vi "test-trajectory-json.vi"(8 "error in (no error)":errorcluster) -> (0 "error out 2":errorcluster, 3 "ALL TESTS PASSED":bool)   [LabVIEW 2019]
uses:
  <vilib>/Rock Robotics/WPI/ThirdParty/JAS_Junk/TrajLib/POSE2D.ctl
  <vilib>/Rock Robotics/WPI/ThirdParty/JAS_Junk/TrajLib/TRANSLATION2D.ctl
  <vilib>/Rock Robotics/WPI/ThirdParty/JAS_Junk/TrajLib/ROTATION2D.ctl
  <vilib>/Rock Robotics/WPI/ThirdParty/JAS_Junk/TrajLib/TRAJECTORY.ctl
  <vilib>/Rock Robotics/WPI/ThirdParty/JAS_Junk/TrajLib/TRAJ_STATE.ctl
  <vilib>/Rock Robotics/SystemInterfaces/NetworkCommunication/NetComm_UsageReport_report.vi
  <vilib>/Rock Robotics/WPI/ThirdParty/JAS_Junk/TrajLib/DiffDriveKinematicsConstraint_New.vi
  TrajectoryState_AlmostEquals.vi
  <vilib>/Rock Robotics/WPI/ThirdParty/JAS_Junk/TrajLib/Util_ApproxEquals.vi
  Pose_AlmostEquals.vi
  Translation_AlmostEquals.vi
  Rotation_AlmostEquals.vi
  <vilib>/Rock Robotics/WPI/ThirdParty/JAS_Junk/TrajLib/Util_CalcDist.vi
  <vilib>/Rock Robotics/WPI/ThirdParty/JAS_Junk/TrajLib/Util_LibraryGlobals.vi
  <vilib>/Rock Robotics/WPI/ThirdParty/JAS_Junk/TrajLib/Trajectory_Library.lvlib
panel:
  out "Read Full \nFilename":string
  out "Write Full \nFilename":string
  in  "Tolerance":dbl=1e-06 format="%#_13g"
  out "outTRAJECTORY":T1 {"States"."POSE"."ROTATION"."SIN" format="%13.4f"; "States"."POSE"."ROTATION"."COS" format="%13.4f"; "States"."POSE"."ROTATION"."VALUE" format="%13.4f"; "States"."POSE"."TRANSLATION"."Y" format="%14.3f"; "States"."POSE"."TRANSLATION"."X" format="%14.3f"; "TotalTImeSecs" format="%20.3f"}
  out "TRAJECTORY":T1 {"States"."POSE"."ROTATION"."SIN" format="%13.4f"; "States"."POSE"."ROTATION"."COS" format="%13.4f"; "States"."POSE"."ROTATION"."VALUE" format="%13.4f"; "States"."POSE"."TRANSLATION"."Y" format="%14.3f"; "States"."POSE"."TRANSLATION"."X" format="%14.3f"; "TotalTImeSecs" format="%20.3f"}
  out "Equals":bool
  out "Read JSON":errorcluster
  out "Create JSON":errorcluster
  out "Waypoints":T3[](array[typedef]) {"ROTATION"."SIN" format="%13.4f"; "ROTATION"."COS" format="%13.4f"; "ROTATION"."VALUE" format="%13.4f"; "TRANSLATION"."Y" format="%14.3f"; "TRANSLATION"."X" format="%14.3f"}
  out "error out":errorcluster
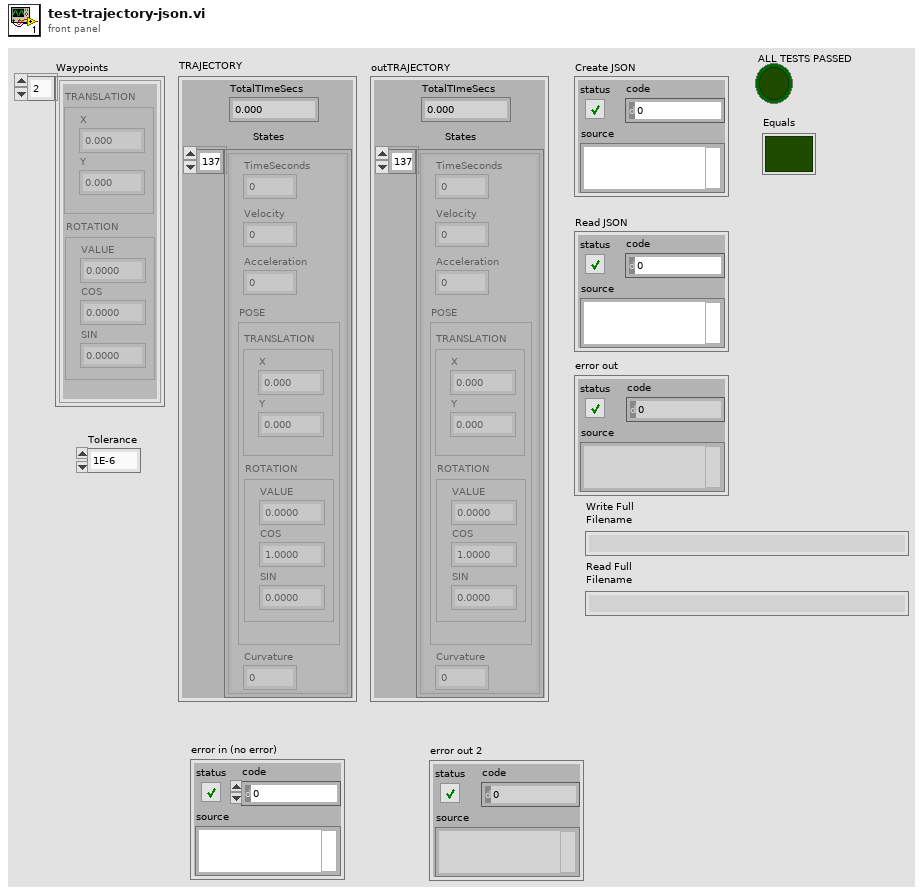
[diagram p1: front panel]
types:
  T1 = typedef "Trajectory_Library.lvlib/TRAJECTORY.ctl" = cluster{"TotalTImeSecs":dbl, "States":T2[]}
  T2 = typedef "Trajectory_Library.lvlib/TRAJ_STATE.ctl" = cluster{"TimeSeconds":dbl, "Velocity":dbl, "Acceleration":dbl, "POSE":T3, "Curvature":dbl}
  T3 = typedef "Trajectory_Library.lvlib/POSE2D.ctl" = cluster{"TRANSLATION":T4, "ROTATION":T5}
  T4 = typedef "Trajectory_Library.lvlib/TRANSLATION2D.ctl" = cluster{"X":dbl, "Y":dbl}
  T5 = typedef "Trajectory_Library.lvlib/ROTATION2D.ctl" = cluster{"VALUE":dbl, "COS":dbl, "SIN":dbl}
  T6 = typedef "Trajectory_Library.lvlib/DIFF_DRIVE_KINEMATICS.ctl" = cluster{"TrackWidth_Meters":dbl}
  T7 = typedef "Trajectory_Library.lvlib/TRAJ_CONFIG.ctl" = cluster{"MaxVelocity":dbl, "Max Acceleration":dbl, "StartVelocity":dbl, "End Velocity":dbl, "Reversed":bool, "DiffDrKineConstntDefined":bool, "CentAcellConstntDefined":bool, "DiffDrVoltConstntDefined":bool, "DIFF_DRIVE_KINE_CONSTRAINT":T8, "CENTRIPETAL_ACCEL_CONSTRAINT":T9, "SwerveDrKineConstntDefined":bool, "SWERVE_DRIVE_KINE_CONSTRAINT":T10, "DIFF_DRIVE_VOLTAGE_CONSTRAINT":T13, "MECANUM_DRIVE_KINE_CONSTRAINT":T15, "MecanumDrKineConstntDefined":bool}
  T8 = typedef "Trajectory_Library.lvlib/TRAJ_CONSTRAINT_DIIF_DRIVE_KINEMATICS.ctl" = cluster{"Max Speed (M/S)":dbl, "DIFF_DRIVE_KINEMATICS":T6, "Max Accel (M/S2)":dbl}
  T9 = typedef "Trajectory_Library.lvlib/TRAJ_CONSTRAINT_CENTRIPETAL_ACCEL.ctl" = cluster{"Max Cent Accel":dbl}
  T10 = typedef "Trajectory_Library.lvlib/TRAJ_CONSTRAINT_SWERVE_DRIVE_KINEMATICS.ctl" = cluster{"Max Speed (M/S)":dbl, "SwerveKinematics":T11}
  T11 = typedef "Trajectory_Library.lvlib/SWERVE_DRIVE_KINEMATICS.ctl" = cluster{"NumModules":i32, "InverseKinematics":T12, "ForwardKinematics":T12, "Modules":T4[], "PrevCoR":T4}
  T12 = typedef "NI_Matrix.lvlib/RealMatrix.ctl" = dbl[][]
  T13 = typedef "Trajectory_Library.lvlib/TRAJ_CONSTRAINT_DIIF_DRIVE_VOLTAGE.ctl" = cluster{"Max Voltage":dbl, "DIFF_DRIVE_KINEMATICS":T6, "SIMPLE_MOTOR_FF":T14}
  T14 = typedef "Trajectory_Library.lvlib/SIMPLE_MOTOR_FF.ctl" = cluster{"Ks":dbl, "Kv":dbl, "Ka":dbl}
  T15 = typedef "Trajectory_Library.lvlib/TRAJ_CONSTRAINT_MECA_DRIVE_KINEMATICS.ctl" = cluster{"Max Speed (M/S)":dbl, "MECA_DRIVE_KINEMATICS":T16}
  T16 = typedef "Trajectory_Library.lvlib/MECA_DRIVE_KINEMATICS.ctl" = cluster{"FrontLeft":T4, "FrontRight":T4, "RearLeft":T4, "RearRight":T4, "InverseKinematics":T12, "ForwardKinematics":T12, "PrevCoR":T4}
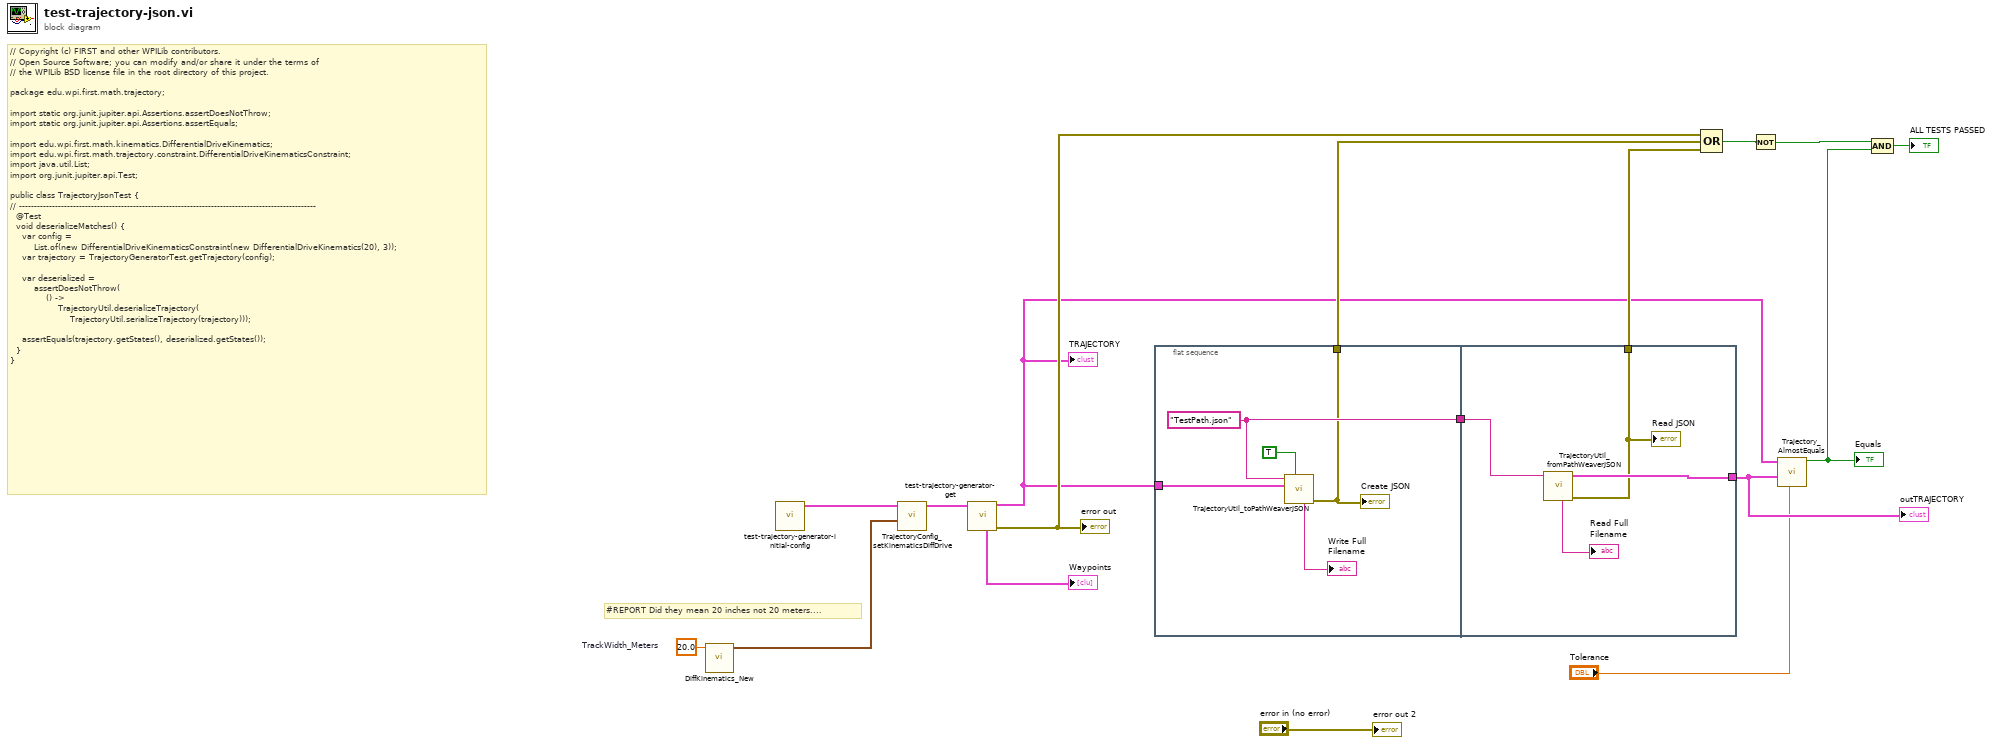
[diagram p0: block diagram]
diagram:
  w16 = 20.0  # TrackWidth_Meters
  # "#REPORT Did they mean 20 inches not 20 meters...."
  # "// Copyright (c) FIRST and other WPILib contributors.\n// Open Source Software; you can modify and/or share it under the terms of\n// the WPILib BSD license file in the root directory of this project.\n\npackage edu.wpi.first.math.trajectory;\n\nimport static org.junit.jupiter.api.Assertions.assertDoesNotThrow;\nimport static org.junit.jupiter.api.Assertions.assertEquals;\n\nimport edu.wpi.first.math.kinematics.DifferentialDriveKinematics;\nimport edu.wpi.first.math.trajectory.constraint.DifferentialDriveKinematicsConstraint;\nimport java.util.List;\nimport org.junit.jupiter.api.Test;\n\npublic class TrajectoryJsonTest {\n// ---------------------------------------------------------------------------------------------------\n  @Test\n  void deserializeMatches() {\n    var config =\n        List.of(new DifferentialDriveKinematicsConstraint(new DifferentialDriveKinematics(20), 3));\n    var trajectory = TrajectoryGeneratorTest.getTrajectory(config);\n\n    var deserialized =\n        assertDoesNotThrow(\n            () ->\n                TrajectoryUtil.deserializeTrajectory(\n                    TrajectoryUtil.serializeTrajectory(trajectory)));\n\n    assertEquals(trajectory.getStates(), deserialized.getStates());\n  }\n}"
  n1 = call <vilib>:"DiffKinematics_New.vi"("TrackWidth_Meters"=w16) -> ("DIFF_DRIVE_KINEMATICS"=w14:T6)  [unwired: 10 in]
  n2 = call "test-trajectory-generator-initial-config.vi"() -> ("traj_config"=w15:T7)  [unwired: 11 in]
  n3 = call <vilib>:"TrajectoryConfig_setKinematicsDiffDrive.vi"("DIFF_DRIVE_KINEMATICS"=w14, "inTRAJECTORY_CONFIG"=w15) -> ("outTRAJECTORY_CONFIG"=w13:T7)  [unwired: 9 in]
  n4 = call "test-trajectory-generator-get.vi"("traj_config"=w13) -> ("error out"=w10:errorcluster, "TRAJECTORY"=w3:T1, "Waypoints"=→"Waypoints":T3[])  [unwired: 8 in]
  "error out" <- w10
  "TRAJECTORY" <- w3
  n5 = flat-sequence {
    tunnel: w3 -> [w22]
    tunnel: [w21] -> w12
    tunnel: [w20] -> w9
    tunnel: w12 -> [w25]
    tunnel: [w26] -> w11
    tunnel: [w24] -> w8
    frame #0 {
      w21 = "TestPath.json" ("FileName")
      n6 = call <vilib>:"TrajectoryUtil_toPathWeaverJSON.vi"("AlwaysOverWrite"=TRUE, "inTRAJECTORY"=w22, "FileName"=w21) -> ("error out"=w20:errorcluster, "Full Filename"=→"Write Full \nFilename":string)  [unwired: 7 in]
      "Create JSON" <- w20
    }
    frame #1 {
      n7 = call <vilib>:"TrajectoryUtil_fromPathWeaverJSON.vi"("FileName"=w25) -> ("error out"=w24:errorcluster, "outTRAJECTORY"=w26:T1, "Full Filename"=→"Read Full \nFilename":string)  [unwired: 8 in]
      "Read JSON" <- w24
    }
  }
  n8 = Compound Arithmetic op=OR(w10, w9, w8) -> (w7:bool)
  n9 = Not(x=w7) -> (.not. x?=w6:bool)
  n10 = call "Trajectory_AlmostEquals.vi"("Tolerance"="Tolerance", "other TRAJECTORY"=w11, "TRAJECTORY"=w3) -> ("Equals"=w5:bool)  [unwired: 8 in]
  "Equals" <- w5
  n11 = Compound Arithmetic op=AND(w6, w5) -> (→"ALL TESTS PASSED":bool)
  "outTRAJECTORY" <- w11
  "error out 2" <- "error in (no error)"
